vi "Scanner Name to Scanner List Item.vi"(3 "Scanner Name":string) -> (0 "Scanner List Item Integer":u16, 1 "Scanner List Item":T1)   [LabVIEW 2017, in "Scan Driver.lvclass"]
uses:
  Scan Driver.lvclass
  Scanner List.ctl
  <vilib>/Utility/error.llb/DialogType.ctl
panel:
  in  "Scanner List.ctl":T1
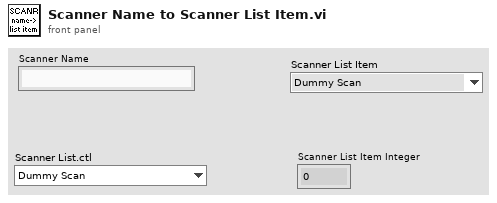
[diagram p1: front panel]
types:
  T1 = typedef "Scan Driver.lvclass/Scanner List.ctl" = enum16{"Dummy Scan", "Analog Output Scan", "Function Gen Scan", "Magnetic Field Lakeshore", "Magnetic Field Lakeshore Continuous", "Magnetic Field Oxford", "Magnetic Field Oxford Continuous", "Magna Current Scan", "Magna Voltage Scan", "Microwave Freq Scan", "Pulse Gen Scan", "Pulse Gen Basic Scan", "Translation Stage Dual", "Translation Stage Coarse", "Translation Stage Fine", "Wavelength Triax 550", "Wavelength Digikröm", "Wavelength ActiveX", "None"}
  T2 = typedef "DialogType.ctl" = u16
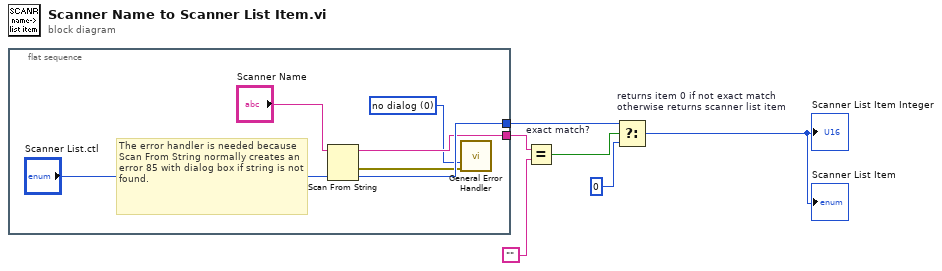
[diagram p0: block diagram]
diagram:
  n1 = flat-sequence {
    tunnel: [w12] -> w5
    tunnel: [w11] -> w3
    frame #0 {
      w7 = T2 0 items=["no dialog", "OK message", "continue or stop message", "OK message + warnings", "continue/stop + warnings"] ("type of dialog (OK msg:1)")
      # "The error handler is needed because Scan From String normally creates an error 85 with dialog box if string is not found."
      n2 = Scan From String "Scan From String"(input string="Scanner Name", default 1="Scanner List.ctl") -> (remaining string=w11:string, error out=w10:errorcluster, output 1=w12:T1)  [unwired: 3 in, 1 out]
      n3 = call <vilib>:"General Error Handler.vi"("type of dialog (OK msg:1)"=w7, "error in (no error)"=w10) -> ()  [unwired: 9 in, 5 out]
    }
  }
  n4 = Equal? "exact match?"(x=w3, y="") -> (x = y?=w4:bool)
  n5 = Select "returns item 0 if not exact match\notherwise returns scanner list item"(t=w5, s=w4, f=u16 0) -> (s? t:f=→"Scanner List Item Integer" →"Scanner List Item":u16)
